vi "Port_Names.vi"() -> ()   [LabVIEW 2010]
uses:
  Anemometry/Anemometry Sub Vis/Controls/ok_button.ctl
  <vilib>/Instr/_visa.llb/VISA Find Search Mode.ctl
panel:
  out "return count":u32
  out "return count 2":u32
  out "List of Port Names":string[](array[string])
  out "Message":string
  out "List of Canonical Names":string[](array[string])
  in  "OK":T1
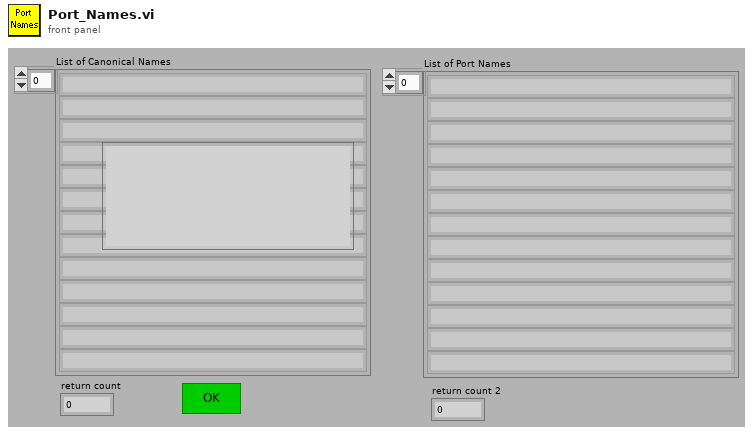
[diagram p1: front panel]
types:
  T1 = typedef "ok_button.ctl" = bool
  T2 = typedef "VISA Find Search Mode.ctl" = u32
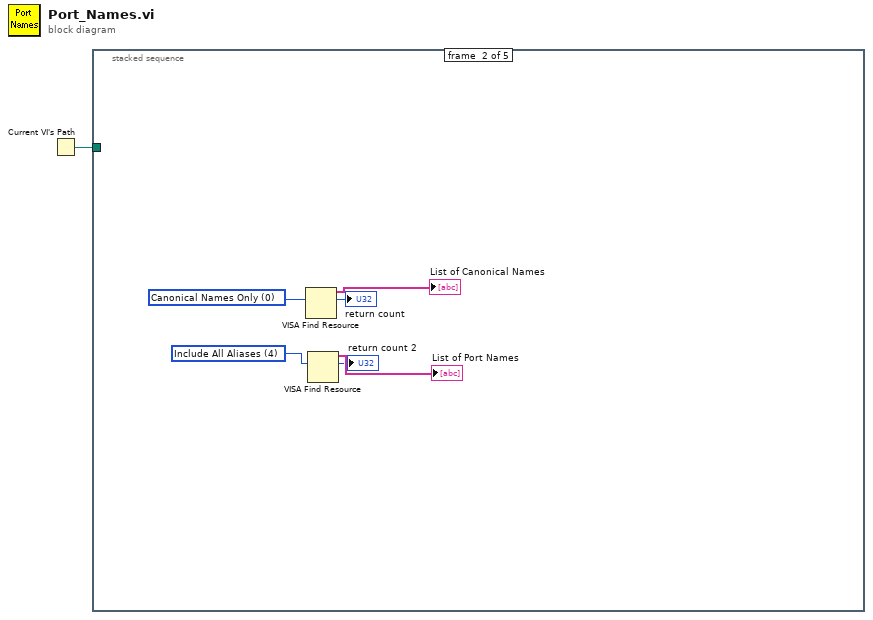
[diagram p0: block diagram]
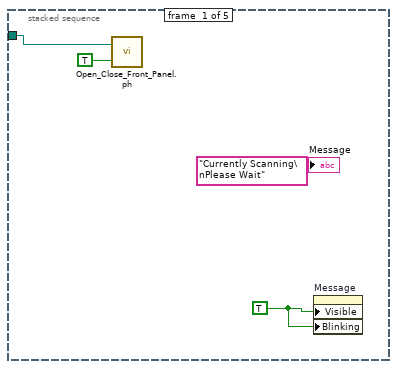
[diagram p2: hidden frame]
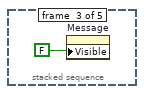
[diagram p3: hidden frame]
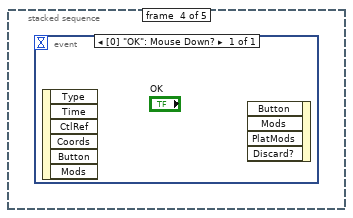
[diagram p4: hidden frame]
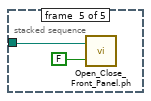
[diagram p5: hidden frame]
diagram:
  n1 = Current VI's Path() -> (path=w1:path)
  n2 = stacked-sequence {
    tunnel: w1 -> [w3 _ _ _ w13]
    frame #0 {
      w2 = TRUE ("Visible")
      n3 = call "Open_Close_Front_Panel.ph.vi"("Front Panel Window:Open"=TRUE, "VI path"=w3) -> ()  [unwired: 2 out]
      n4 = property on="Message" class="Str"("Visible"=w2, "Blinking"=w2) -> ()  [unwired: 2 in, 2 out]
      "Message" <- "Currently Scanning\nPlease Wait" ("Message")
    }
    frame #1 {
      w8 = T2 4 items=["Canonical Names Only"=0, "Aliases Only"=1, "Include Matching Aliases"=2, "Include All Aliases"=4] ("Search Mode")
      w10 = T2 0 items=["Canonical Names Only"=0, "Aliases Only"=1, "Include Matching Aliases"=2, "Include All Aliases"=4] ("Search Mode")
      n5 = VISA Find Resource(10:w10) -> (2:→"return count":u32, 3:→"List of Canonical Names":string[])  [unwired: 1 in, 2 out]
      n6 = VISA Find Resource(10:w8) -> (2:→"return count 2":u32, 3:→"List of Port Names":string[])  [unwired: 2 in, 1 out]
    }
    frame #2 {
      n7 = property on="Message" class="Str"("Visible"=FALSE) -> ()  [unwired: 2 in, 2 out]
    }
    frame #3 {
      n8 = event shown="[0] \"OK\": Mouse Down?" {
        selector: _ -> [_]
        dyn-events: _ -> [_]
        timeout: _ -> [_]
        event Mouse Down? {
          n9 = event-data() -> ()  [unwired: 7 out]
          n10 = event-data() -> ()  [unwired: 1 in, 5 out]
        }
      }
    }
    frame #4 {
      n11 = call "Open_Close_Front_Panel.ph.vi"("Front Panel Window:Open"=FALSE, "VI path"=w13) -> ()  [unwired: 2 out]
    }
  }
